vi "Run Bfr Rx - PingPong - Add to Active.vi"(5 "Data Size in":u64, 7 "Data in":u8[](array[numeric]), 8 "error in (no error)":errorcluster, 11 "Ping Pong Buffer in":T1 {"Active Buffer Ref" format="%016x"}) -> (0 "error out":errorcluster, 3 "Ping Pong Buffer out":T1 {"Active Buffer Ref" format="%016x"})   [LabVIEW 2016, in "UDP-Custom-Device Engine.lvlib"]
uses:
  UDP-Custom-Device Engine.lvlib
  Types/Engine - Buffered Rx Ping Pong Buffer.ctl
  Types/Engine - Buffered Rx Active Buffer.ctl
  <vilib>/NI Veristand/VeriStand Data/Pointer Operations/Pointer.Write (1D U8).vi
  <vilib>/NI Veristand/VeriStand Data/VeriStand Data.lvlib
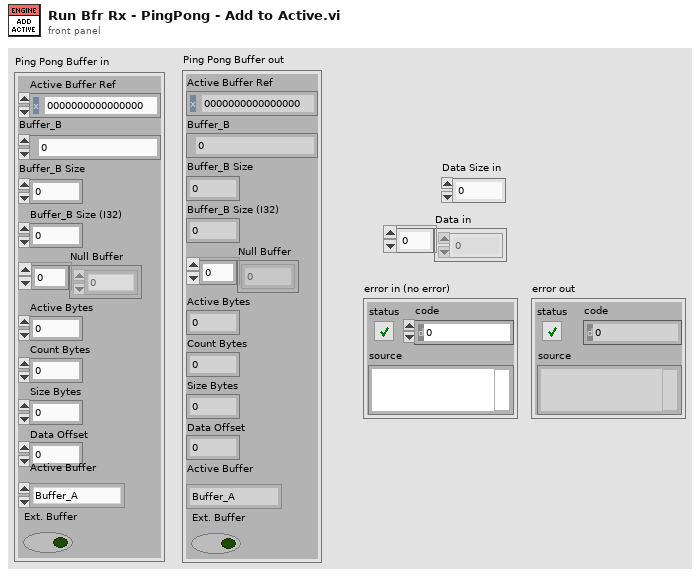
[diagram p1: front panel]
types:
  T1 = typedef "UDP-Custom-Device Engine.lvlib/Engine - Buffered Rx Ping Pong Buffer.ctl" = cluster{"Active Buffer Ref":u64, "Buffer_B":u64, "Buffer_B Size":u64, "Buffer_B Size (I32)":i32, "Null Buffer":u8[], "Active Bytes":u64, "Count Bytes":u64, "Size Bytes":u64, "Data Offset":u64, "Active Buffer":T2, "Ext. Buffer":bool}
  T2 = typedef "UDP-Custom-Device Engine.lvlib/Engine - Buffered Rx Active Buffer.ctl" = enum16{"Buffer_A", "Buffer_B"}
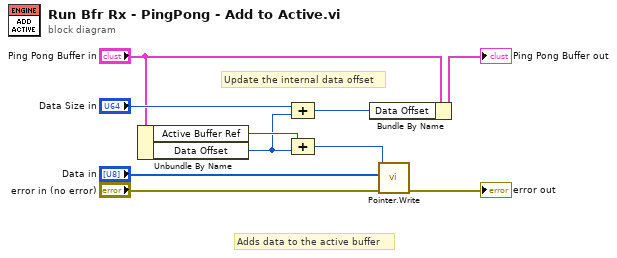
[diagram p0: block diagram]
diagram:
  # "Update the internal data offset"
  # "Adds data to the active buffer"
  n1 = Unbundle By Name("Ping Pong Buffer in") -> ("Active Buffer Ref"=w7:u64, "Data Offset"=w4:u64)
  n2 = Compound Arithmetic op=ADD("Data Size in", w4) -> (w2:u64)
  n3 = Compound Arithmetic op=ADD(w7, w4) -> (w6:u64)
  n4 = Bundle By Name(cluster="Ping Pong Buffer in", "Data Offset"=w2) -> (→"Ping Pong Buffer out":T1)
  n5 = call-poly <vilib>:"Pointer.Write.vi"("error in (no error)"="error in (no error)", "values"="Data in", "pointer in"=w6) -> ("error out"=→"error out":errorcluster)  [unwired: 6 in, 2 out]
